vi "simple_wf_playback.vi"() -> ()   [LabVIEW 2013]
uses:
  <vilib>/Waveform/WDTFileIO.llb/Read Waveform from File.vi
  <vilib>/Waveform/WDTOps.llb/WDT Append Waveforms DBL.vi
panel:
  out "웨이브폼 그래프":waveform(dbl)(graph)
  out "숫자형":i32
  in  "확인 버튼":bool
  out "웨이브폼 차트":waveform(dbl)(graph)
  in  "file path (dialog if empty)":path caption="파일 경로(비었을 경우 대화 상자 창)"
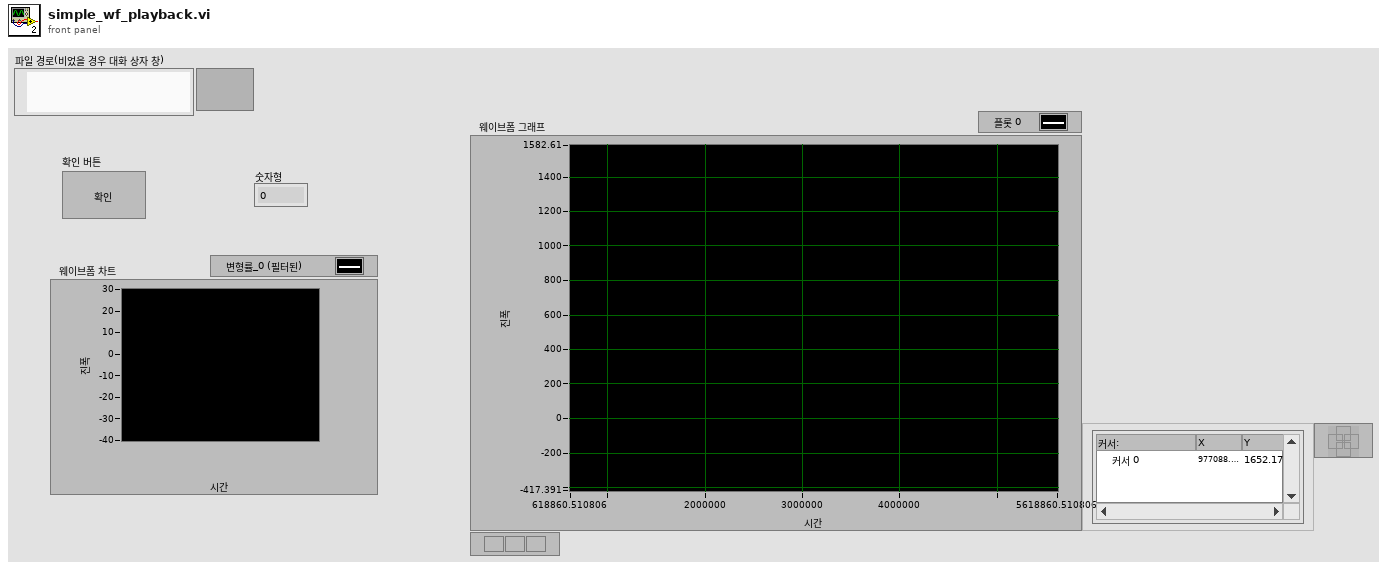
[diagram p1: front panel]
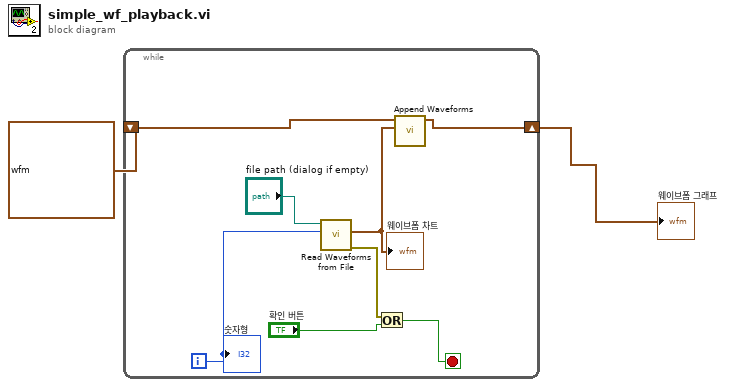
[diagram p0: block diagram]
diagram:
  n1 = while {
    shift-right: [w3] -> w2
    shift-left: waveform(dbl) {"t0"=timestamp(0 s since 1904-01-01), "dt"=1.0, "Y"=[]} ("waveform out") -> [w4]
    i -> [w6]
    stop <- w7 stop-if-true
    n2 = call-poly <vilib>:"Read Waveforms from File.vi"("offset (records:0)"=w6, "file path (dialog if empty)"="file path (dialog if empty)") -> ("error out"=w9:errorcluster, "first waveform in record"=w5:waveform(dbl))  [unwired: 4 in, 2 out]
    "웨이브폼 차트" <- w5
    n3 = Or(x=w9, y="확인 버튼") -> (x .or. y?=w7:bool)
    n4 = call-poly <vilib>:"Append Waveforms.vi"("waveform B"=w5, "waveform A"=w4) -> ("waveform out"=w3:waveform(dbl))  [unwired: 8 in, 1 out]
    "숫자형" <- w6
  }
  "웨이브폼 그래프" <- w2
